vi "continuous_sin.vi"(5 "file path (use dialog)":path, 6 "Amplitude":dbl, 7 "Frequency (MHz)":dbl, 8 "Numeric":i32, 9 "Trigger Width (us)":dbl format="%#_13g", 10 "Pulse Amplitude":dbl=1.4 format="%#_13g", 11 "DAC frequency (MHz)":dbl) -> (2 "output waveform 2":waveform(dbl)(graph), 3 "output waveform":waveform(dbl)(graph))   [LabVIEW 2016]
panel:
  out "Number of Points":i32
  out "x-y":u32
  in  "Pulse Center":dbl format="%#_13g"
  in  "Envelope Decay Time (micro s)":dbl
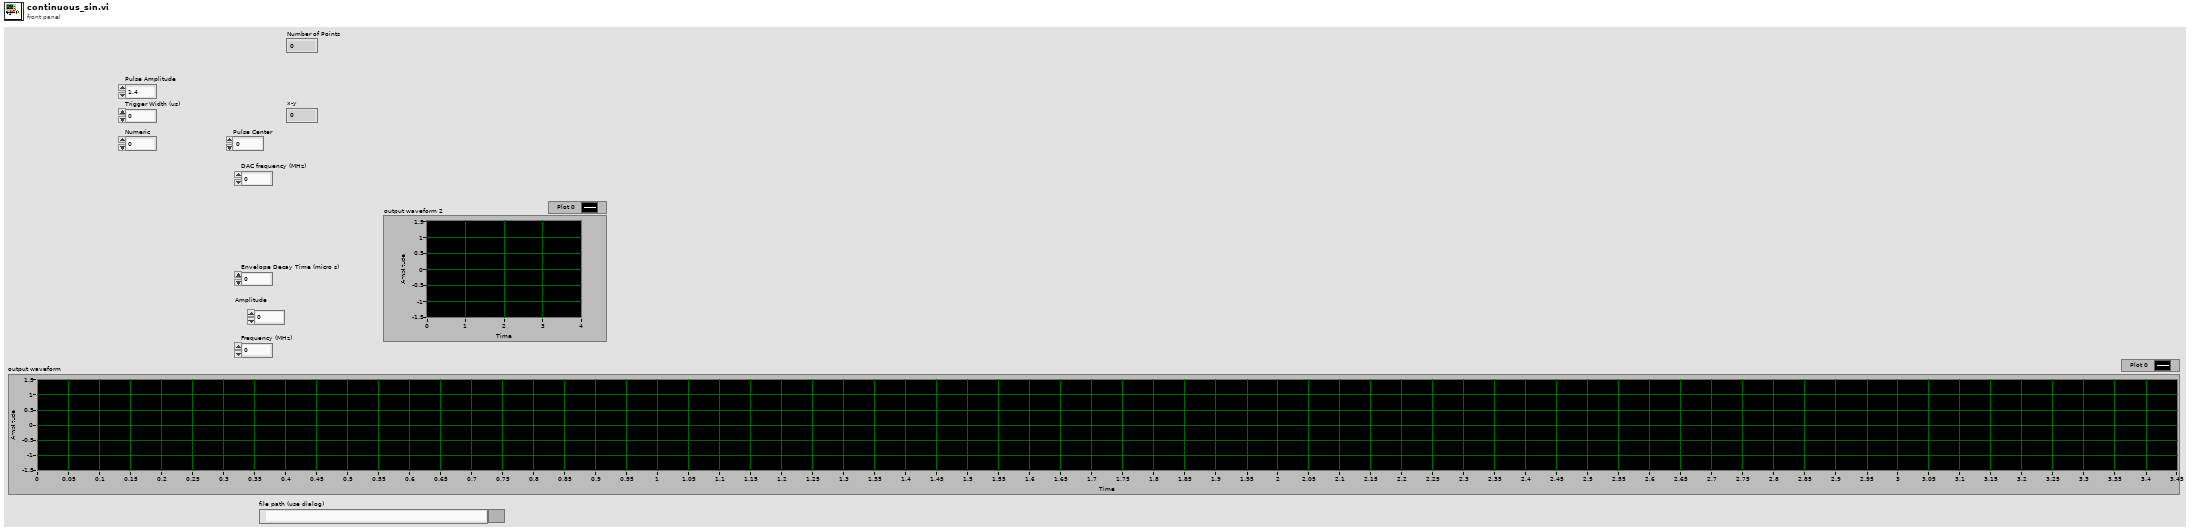
[diagram p1: front panel]
types:
  T1 = enum16{"open", "replace", "create", "open or create", "replace or create", "replace or create with confirmation"}
  T2 = enum16{"big-endian, network order", "native, host order", "little-endian"}
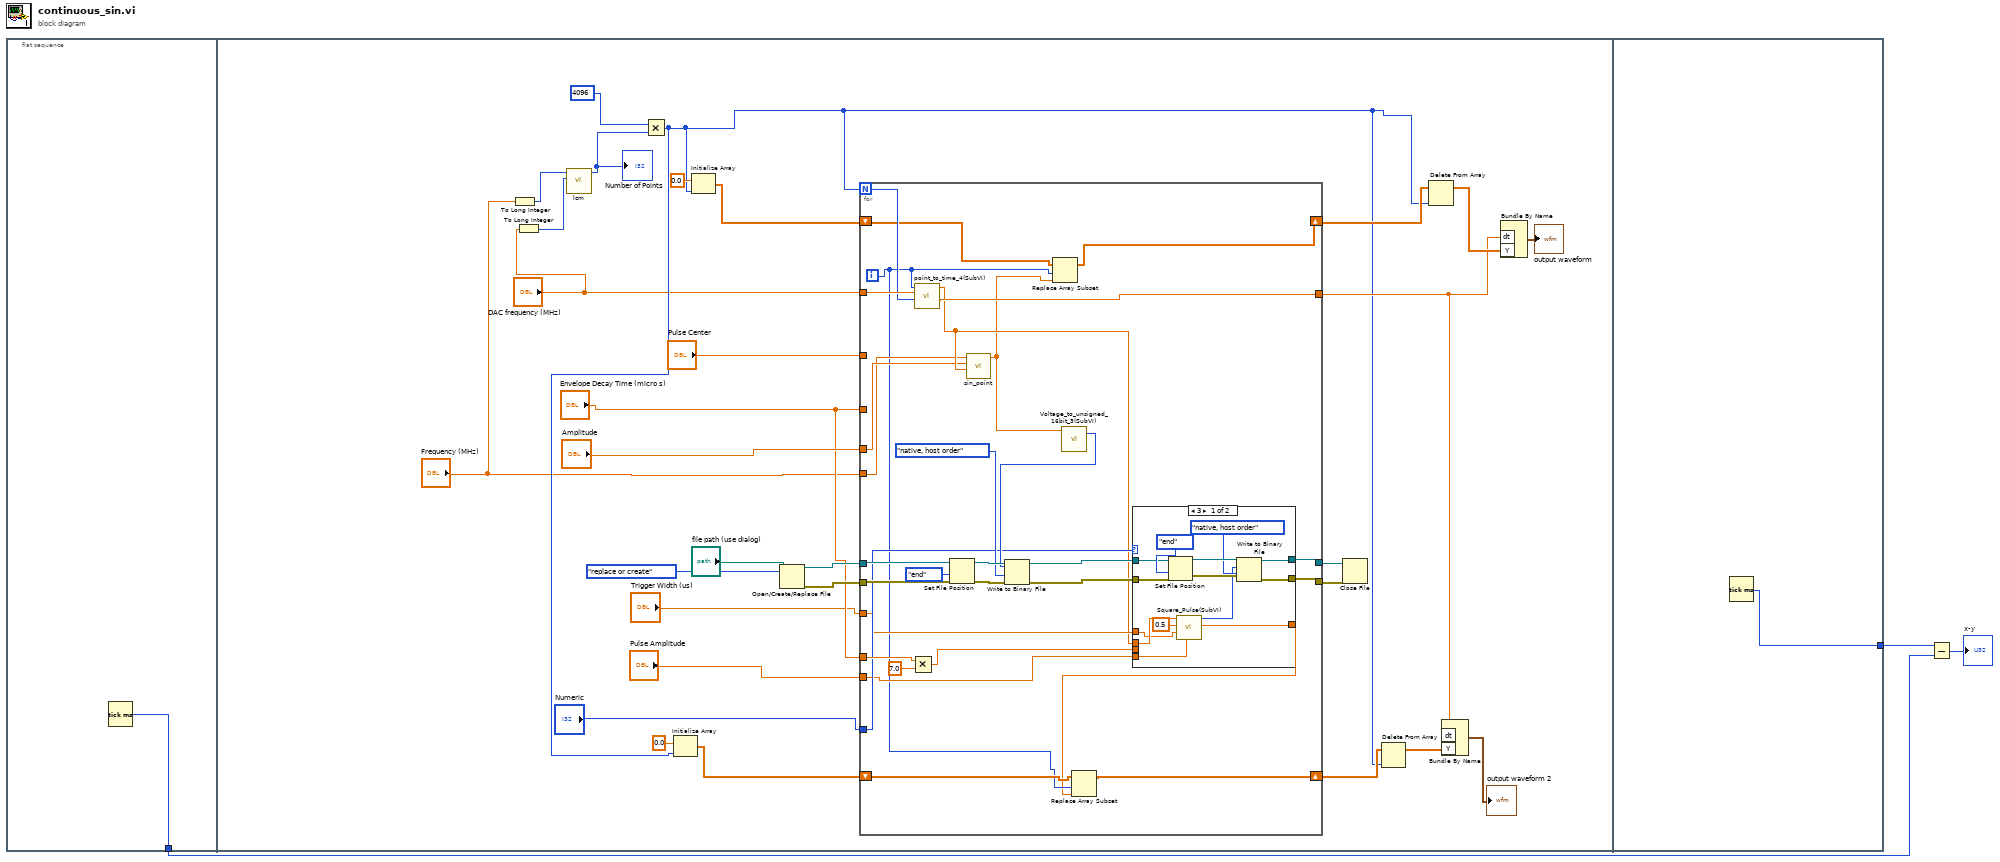
[diagram p0: block diagram]
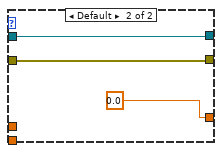
[diagram p2: hidden frame]
diagram:
  n1 = flat-sequence {
    tunnel: [w4] -> w2
    tunnel: [w82] -> w3
    frame #0 {
      n2 = Tick Count (ms)() -> (millisecond timer value=w4:u32)
    }
    frame #1 {
      n3 = To Long Integer(number="Frequency (MHz)") -> (32bit integer=w6:i32)
      n4 = To Long Integer(number="DAC frequency (MHz)") -> (32bit integer=w7:i32)
      n5 = call "lcm.vi"("DAC Frequency"=w7, "Frequency"=w6) -> ("Number of Points"=w9:i32)  [unwired: 9 in]
      "Number of Points" <- w9
      n6 = Multiply(x=4096, y=w9) -> (x*y=w10:i32)
      n7 = Initialize Array(0.0 ("element"), w10) -> (w11:dbl[])
      n8 = Initialize Array(0.0 ("element"), w10) -> (w13:dbl[])
      n9 = Open/Create/Replace File(file path (use dialog)="file path (use dialog)", operation (0:open)=T1."replace or create") -> (refnum out=w30:refnum<file>, error out=w31:errorcluster)  [unwired: 4 in, 1 out]
      n10 = for {
        N: w10 -> [w56]
        tunnel: "Amplitude" -> [w43]
        shift-right: [w40] -> w34
        shift-left: w13 -> [w41]
        tunnel: "Envelope Decay Time (micro s)" -> [_]
        tunnel: "Frequency (MHz)" -> [w42]
        tunnel: "DAC frequency (MHz)" -> [w57]
        tunnel: [w55] -> w17
        tunnel: w30 -> [w64]
        tunnel: w31 -> [w63]
        tunnel: [w48] -> w32
        tunnel: [w47] -> w33
        tunnel: "Pulse Center" -> [_]
        tunnel: "Pulse Amplitude" -> [w51]
        tunnel: "Envelope Decay Time (micro s)" -> [w54]
        shift-right: [w35] -> w18
        shift-left: w11 -> [w38]
        tunnel: "Numeric" -> [w52]
        tunnel: "Trigger Width (us)" -> [w45]
        i -> [w37]
        n11 = Multiply(x=w54, y=7.0) -> (x*y=w50:dbl)
        n12 = call "point_to_time_4(SubVI).vi"("number of points"=w56, "DAC frequency(MHz)"=w57, "point location"=w37) -> ("dt (us)"=w55:dbl, "time (us)"=w44:dbl)  [unwired: 6 in, 1 out]
        n13 = Set File Position(refnum=w64, from (0:start)=enum16{"start", "end", "current"}."end", error in=w63) -> (refnum out=w62:refnum<file>, error out=w61:errorcluster)  [unwired: 1 in]
        n14 = call "sin_point.vi"("Time"=w44, "Amplitude"=w43, "Frequency"=w42) -> ("Output"=w39:dbl)  [unwired: 8 in]
        n15 = Replace Array Subset(array=w41, new element=w39, index=w37) -> (w40:dbl[])
        n16 = call "Voltage_to_unsigned_16bit_3(SubVI).vi"("Voltage_in"=w39) -> ("unsigned 16bit integer"=w58:u16)  [unwired: 10 in]
        n17 = Write to Binary File(file (use dialog)=w62, data=w58, error in=w61, 9:T2."native, host order" ("byte order (0:big-endian, network order)")) -> (refnum out=w46:refnum<file>, error out=w49:errorcluster)  [unwired: 2 in, 1 out]
        n18 = case shown="3" w52 {
          tunnel: w51 -> [w78 _]
          tunnel: [w77 0.0] -> w36
          tunnel: w44 -> [w76 _]
          tunnel: w50 -> [_ _]
          tunnel: w49 -> [w74 w81]
          tunnel: [w71 w80] -> w48
          tunnel: [w70 w81] -> w47
          tunnel: w46 -> [w67 w80]
          tunnel: w45 -> [w65 _]
          frame 3 {
            n19 = Set File Position(refnum=w67, from (0:start)=enum16{"start", "end", "current"}."end", error in=w74) -> (refnum out=w73:refnum<file>, error out=w72:errorcluster)  [unwired: 1 in]
            n20 = call "Square_Pulse(SubVI).vi"("High Voltage (V)"=w78, "Pulse Width"=w65, "Pulse Start (us)"=0.5, "Time"=w76) -> ("Voltage Out"=w77:dbl, "unsigned 16-bit out"=w68:u16)  [unwired: 6 in]
            n21 = Write to Binary File(file (use dialog)=w73, data=w68, error in=w72, 9:T2."native, host order" ("byte order (0:big-endian, network order)")) -> (refnum out=w71:refnum<file>, error out=w70:errorcluster)  [unwired: 2 in, 1 out]
          }
          frame Default {
          }
        }
        n22 = Replace Array Subset(array=w38, new element=w36, index=w37) -> (w35:dbl[])
      }
      n23 = Close File(refnum=w32, error in=w33) -> ()  [unwired: 2 out]
      n24 = Delete From Array(array=w18, index=w10) -> (array with subset deleted=w20:dbl[])  [unwired: 1 in, 1 out]
      n25 = Delete From Array(array=w34, index=w10) -> (array with subset deleted=w27:dbl[])  [unwired: 1 in, 1 out]
      n26 = Bundle By Name("dt"=w17, "Y"=w20) -> (→"output waveform 2":waveform(dbl))  [unwired: 1 in]
      n27 = Bundle By Name("dt"=w17, "Y"=w27) -> (→"output waveform":waveform(dbl))  [unwired: 1 in]
    }
    frame #2 {
      n28 = Tick Count (ms)() -> (millisecond timer value=w82:u32)
    }
  }
  n29 = Subtract(x=w3, y=w2) -> (x-y=→"x-y":u32)
